vi "ini.vi"(8 "error in (no error)":errorcluster) -> (0 "error out":errorcluster, 2 "Queue Cluster":T1)   [LabVIEW 2017]
uses:
  Ctl/MEMS.ctl
  ModbusRTU/ModbusRTUCmd.ctl
  ModbusRTU/Process/Process.ctl
  ModbusRTU/Caculator/Caculator.ctl
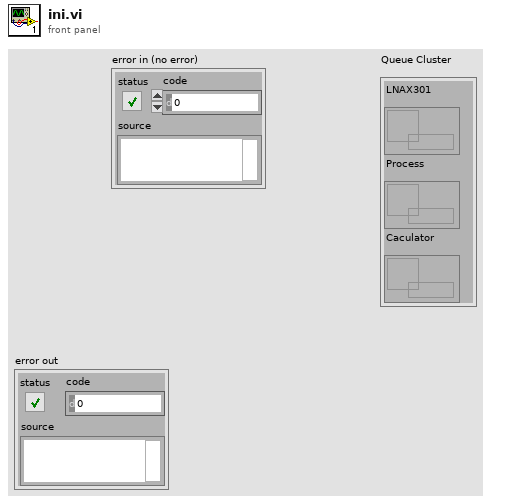
[diagram p1: front panel]
types:
  T1 = typedef "MEMS.ctl" = cluster{"LNAX301":refnum<queue>, "Process":refnum<queue>, "Caculator":refnum<queue>}
  T2 = typedef "Caculator.ctl" = cluster{"cmd":enum16{"Idle", "ini", "Disconnect", "UpdateSetup", "ChangeView", "Caculator", "Exit"}, "Var":variant}
  T3 = typedef "Process.ctl" = cluster{"cmd":enum16{"Idle", "ini", "CheckData", "Disconnect", "UpdateSetup", "UpdateInstance", "Exit"}, "Var":variant}
  T4 = typedef "ModbusRTUCmd.ctl" = cluster{"CMD":enum16{"Idle", "ini", "Connect", "Setup", "Read", "Disconnect", "Exit"}, "Var":variant}
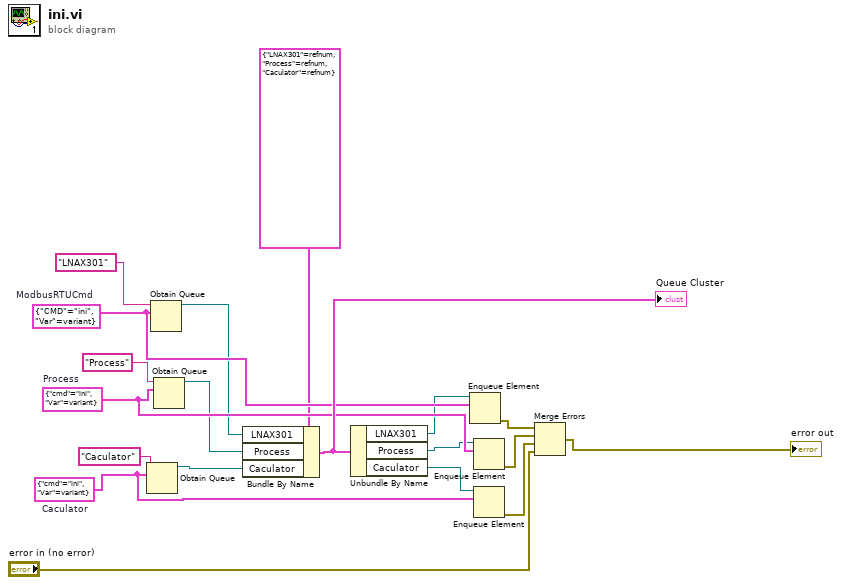
[diagram p0: block diagram]
diagram:
  w15 = T2 {"cmd"=enum."ini", "Var"=variant}  # Caculator
  w14 = T3 {"cmd"=enum."ini", "Var"=variant}  # Process
  w13 = T4 {"CMD"=enum."ini", "Var"=variant}  # ModbusRTUCmd
  n1 = Obtain Queue(name (unnamed)="Caculator", element data type=w15) -> (queue out=w9:refnum<queue>)  [unwired: 3 in, 2 out]
  n2 = Obtain Queue(name (unnamed)="LNAX301", element data type=w13) -> (queue out=w7:refnum<queue>)  [unwired: 3 in, 2 out]
  n3 = Obtain Queue(name (unnamed)="Process", element data type=w14) -> (queue out=w8:refnum<queue>)  [unwired: 3 in, 2 out]
  n4 = Bundle By Name(cluster=T1 {"LNAX301"=refnum, "Process"=refnum, "Caculator"=refnum}, "LNAX301"=w7, "Process"=w8, "Caculator"=w9) -> (w19:T1)
  "Queue Cluster" <- w19
  n5 = Unbundle By Name(w19) -> ("LNAX301"=w10:refnum<queue>, "Process"=w11:refnum<queue>, "Caculator"=w12:refnum<queue>)
  n6 = Enqueue Element(queue=w10, element=w13) -> (error out=w16:errorcluster)  [unwired: 2 in, 2 out]
  n7 = Enqueue Element(queue=w11, element=w14) -> (error out=w17:errorcluster)  [unwired: 2 in, 2 out]
  n8 = Enqueue Element(queue=w12, element=w15) -> (error out=w18:errorcluster)  [unwired: 2 in, 2 out]
  n9 = Merge Errors(w16, w17, w18, "error in (no error)") -> (→"error out":errorcluster)
